vi "replace_head.vi"(7 "save":bool=TRUE, 9 "datatype":string, 11 "nii_source":path) -> ()   [LabVIEW 2014]
uses:
  nii_read_head.vi
  nii_write.vi
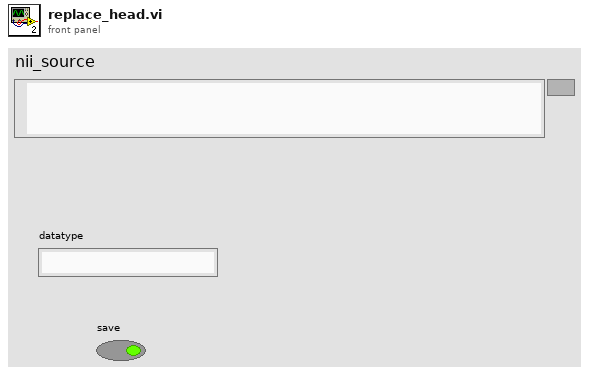
[diagram p1: front panel]
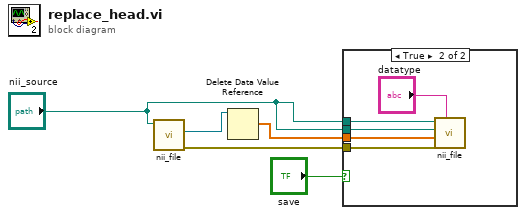
[diagram p0: block diagram]
diagram:
  n1 = call-poly "nii_file.vi"("file (use dialog)"="nii_source") -> ("error out"=w5:errorcluster, "data value reference"=w3:refnum<data-value>)  [unwired: 6 in, 3 out]
  n2 = Delete Data Value Reference(data value reference=w3) -> (data value=w2:cdb[])  [unwired: 1 in, 1 out]
  n3 = case shown="True" "save" {
    tunnel: "nii_source" -> [_ w10]
    tunnel: w5 -> [_ w9]
    tunnel: "nii_source" -> [_ w8]
    tunnel: w2 -> [_ w6]
    frame False {
    }
    frame True {
      n4 = call-poly "nii_file.vi"("datatype"="datatype", "error in (no error)"=w9, "data in"=w6, "nii_write"=w8, "nii_source"=w10) -> ()  [unwired: 6 in, 1 out]
    }
  }
